vi "Get All Subaddress Sections.vi"(8 "error in":errorcluster, 11 "remote terminal":T1 format="%.0x") -> (0 "error out":errorcluster, 2 "subaddress sections":T1[](array[typedef]) format="%.0x", 3 "remote terminal out":T1 format="%.0x")   [LabVIEW 2020, in "AIM MIL-STD-1553 Scripting.lvlib"]
doc: "Returns all of the <b>subaddress sections</b> in the <b>remote terminal</b>."
uses:
  AIM MIL-STD-1553 Scripting.lvlib
  <vilib>/NI VeriStand/Custom Device API/Custom Device Item Ref.ctl
  Constants.vi
  <vilib>/NI VeriStand/Custom Device Tools/Custom Device Utility Library/NI VeriStand - Search for All Items by GUID.vi
  <vilib>/NI VeriStand/Custom Device Tools/Custom Device Utility Library/Custom Device Utility Library.lvlib
  <vilib>/NI VeriStand/Custom Device API/Custom Device API.lvlib
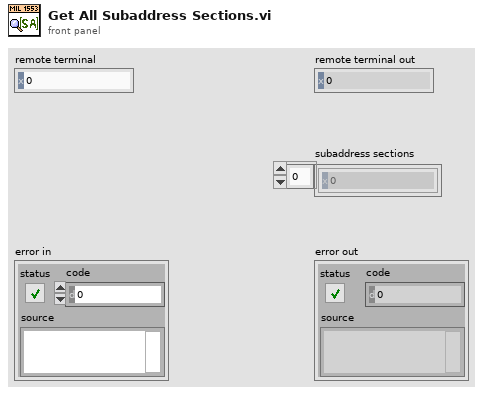
[diagram p1: front panel]
types:
  T1 = typedef "Custom Device API.lvlib/Custom Device Item Ref.ctl" = u64
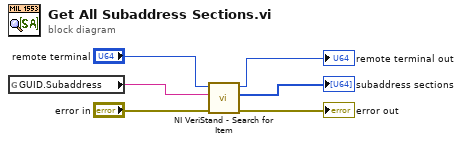
[diagram p0: block diagram]
diagram:
  n1 = global read "Constants.vi" "GUID.Subaddress"() -> (w6:string)
  n2 = call-poly <vilib>:"NI VeriStand - Search for Item.vi"("error in"="error in", "Item GUID"=w6, "Section Ref in"="remote terminal") -> ("error out"=→"error out":errorcluster, "Item Refs"=→"subaddress sections":T1[], "Section Ref out"=→"remote terminal out":T1)  [unwired: 5 in, 1 out]
